vi "05TRM500_AnalyzeReceive_V2.vi"(5 "INC":dbl, 6 "Directory":path, 7 "MPH":dbl, 8 "error in (no error)":errorcluster, 10 "String":string, 11 "Enum":enum16{"Initialize", "Analyze"}(ring)) -> (0 "error out":errorcluster, 3 "Data":T1)   [LabVIEW 2020]
uses:
  <vilib>/regexp/Match Regular Expression.xnode
panel:
  out "File Ref":refnum<file>
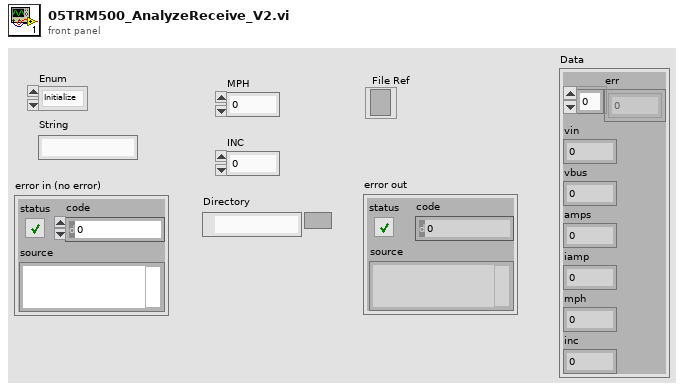
[diagram p1: front panel]
types:
  T1 = cluster{"err":i32[], "vin":i32, "vbus":i32, "amps":i32, "iamp":i32, "mph":i32, "inc":i32}
  T2 = enum16{"Initialize", "Next", "Send RSET", "Set MPH", "Set INC", "Part to 0"}
  T3 = enum16{"Initialize", "FootReceive", "FootDisplay"}
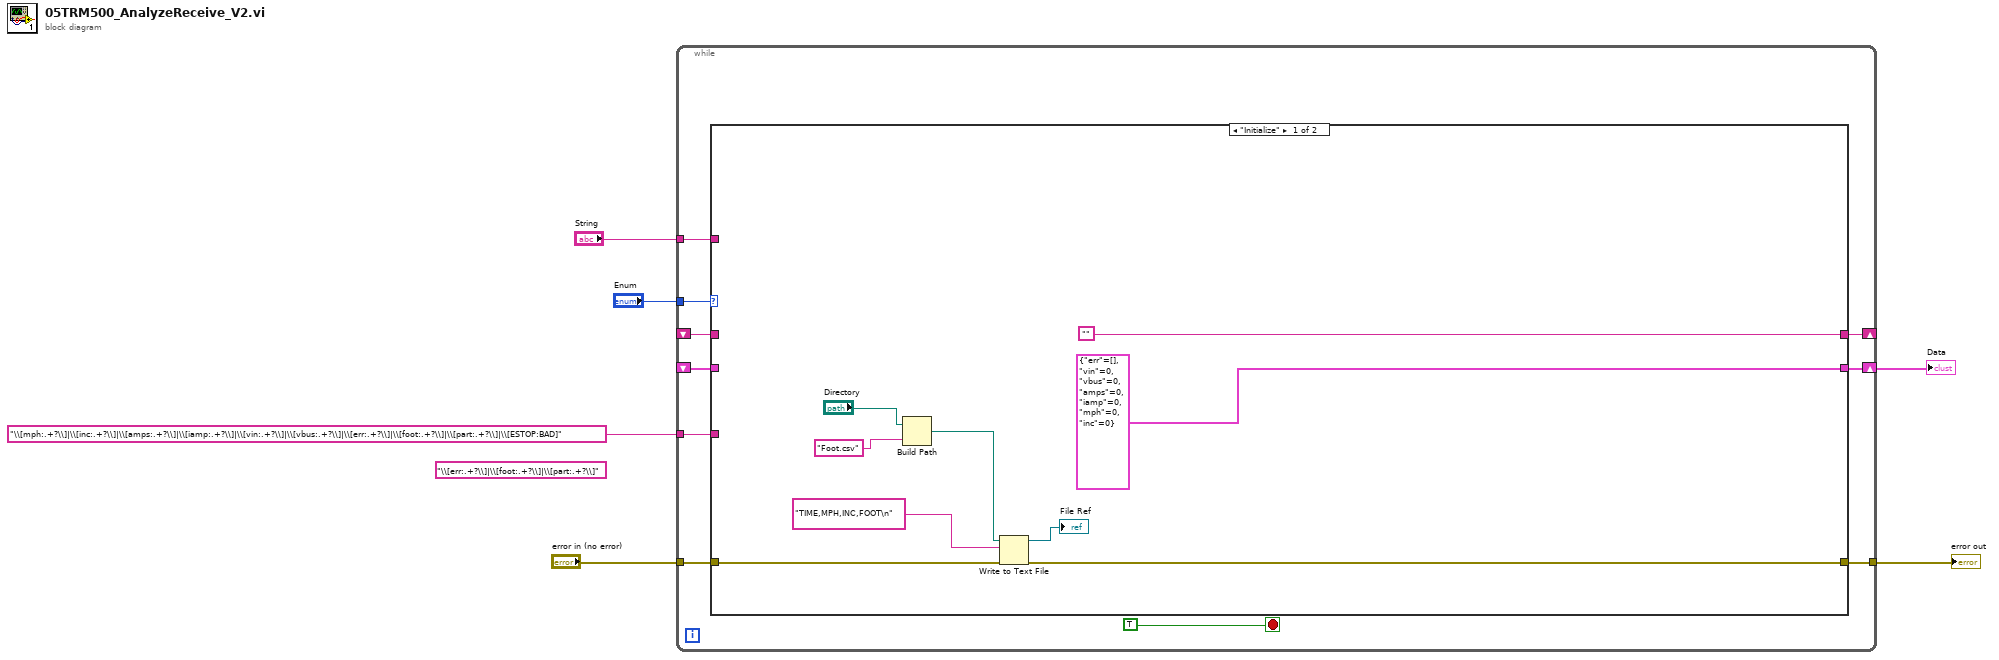
[diagram p0: block diagram]
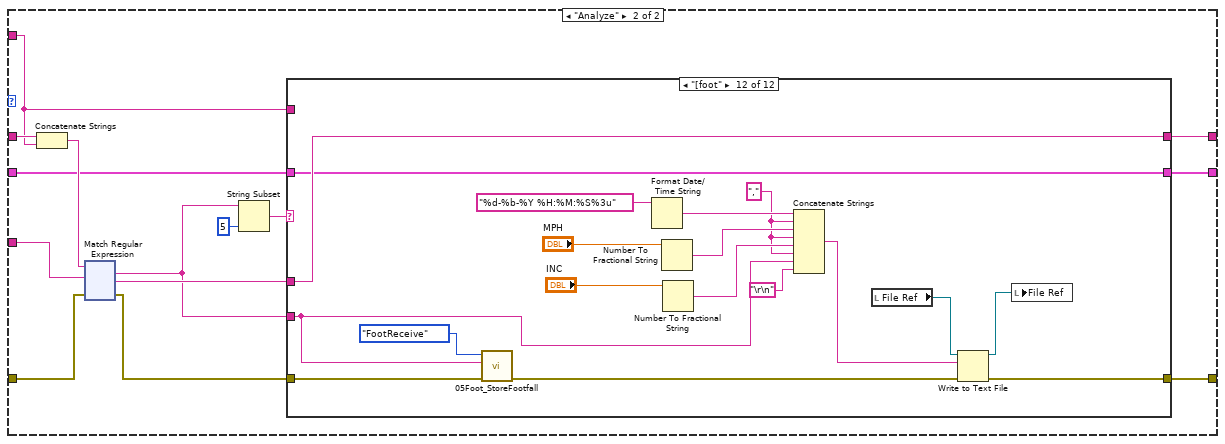
[diagram p2: hidden frame]
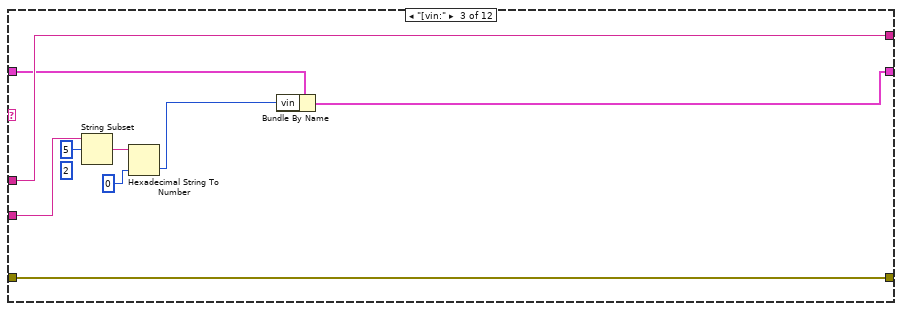
[diagram p5: hidden frame]
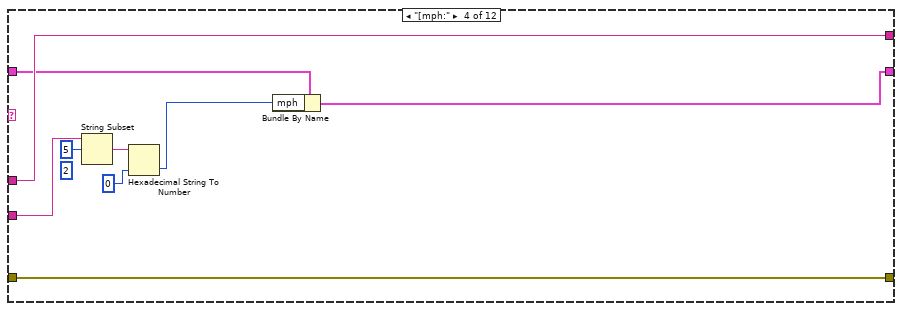
[diagram p6: hidden frame]
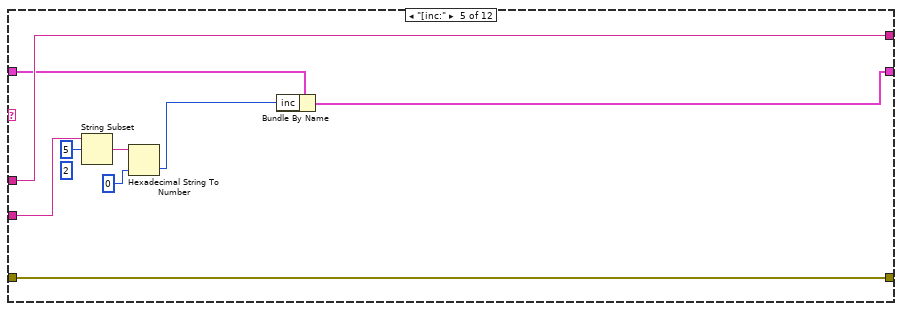
[diagram p7: hidden frame]
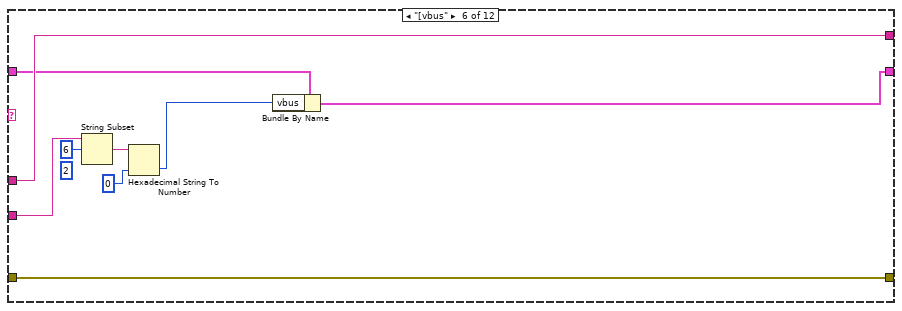
[diagram p8: hidden frame]
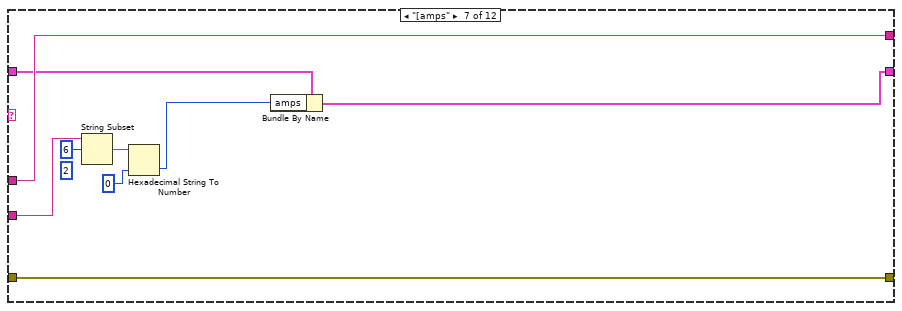
[diagram p9: hidden frame]
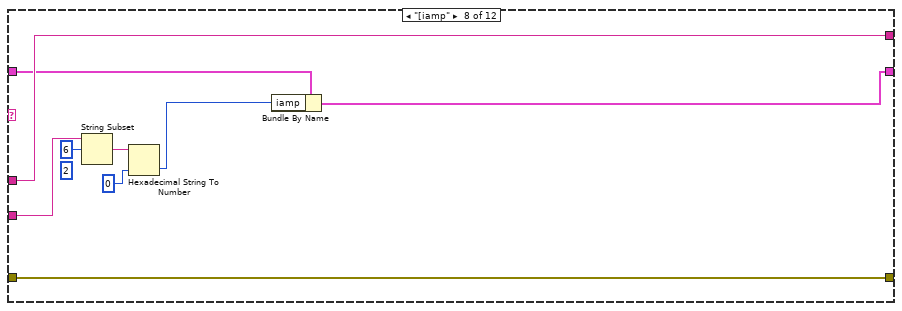
[diagram p10: hidden frame]
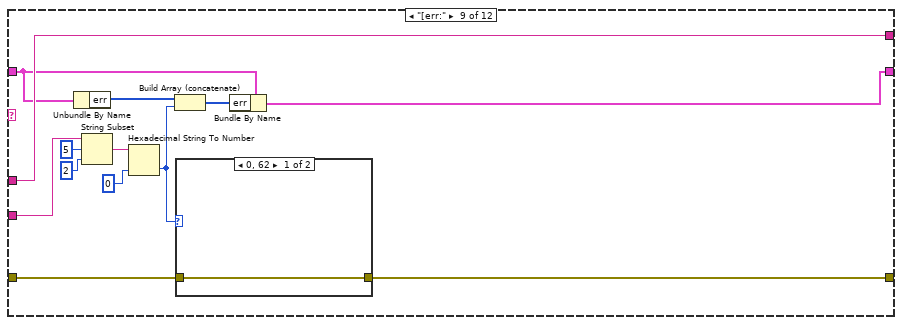
[diagram p11: hidden frame]
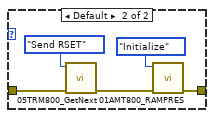
[diagram p12: hidden frame]
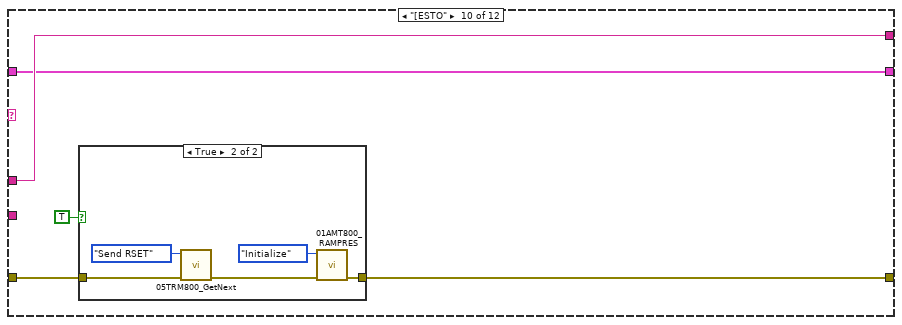
[diagram p13: hidden frame]
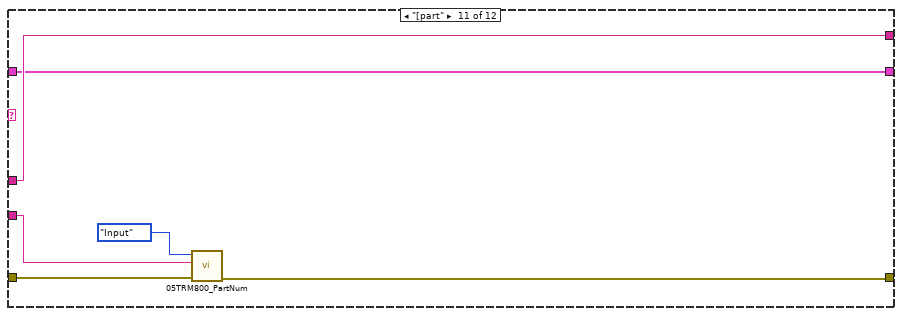
[diagram p15: hidden frame]
diagram:
  (unwired) "\\[err:.+?\\]|\\[foot:.+?\\]|\\[part:.+?\\]" ("regular expression")
  n1 = while {
    tunnel: "error in (no error)" -> [w13]
    tunnel: [w14] -> w5
    tunnel: "Enum" -> [w15]
    shift-right: [w12] -> _
    shift-left: _ -> [w11]
    tunnel: "String" -> [w10]
    tunnel: "\\[mph:.+?\\]|\\[inc:.+?\\]|\\[amps:.+?\\]|\\[iamp:.+?\\]|\\[vin:.+?\\]|\\[vbus:.+?\\]|\\[err:.+?\\]|\\[foot:.+?\\]|\\[part:.+?\\]|\\[ESTOP:BAD]" ("regular expression") -> [w9]
    shift-right: [w8] -> w1
    shift-left: _ -> [w7]
    stop <- TRUE stop-if-true
    n2 = case shown="\"Initialize\"" w15 {
      tunnel: [w20 w35] -> w14
      tunnel: w13 -> [w23 w32]
      tunnel: ["" w37] -> w12
      tunnel: w11 -> [_ w39]
      tunnel: w10 -> [_ w38]
      tunnel: w9 -> [_ w34]
      tunnel: [T1 {"err"=[], "vin"=0, "vbus"=0, "amps"=0, "iamp"=0, "mph"=0, "inc"=0} w26] -> w8
      tunnel: w7 -> [_ w27]
      frame "Initialize" {
        n3 = Build Path(base path="Directory", name or relative path="Foot.csv") -> (appended path=w17:path)
        n4 = Write to Text File(file (use dialog)=w17, text="TIME,MPH,INC,FOOT\n", error in=w23) -> (refnum out=→"File Ref":refnum<file>, error out=w20:errorcluster)  [unwired: 1 in, 1 out]
      }
      frame "Analyze" {
        n5 = Concatenate Strings(w39, w38) -> (w33:string)
        n6 = xnode "Match Regular Expression"("input string"=w33, "regular expression"=w34, "error in"=w32) -> ("whole match"=w28:string, "after match"=w36:string, "error out"=w31:errorcluster)  [unwired: 3 in, 2 out]
        n7 = String Subset(string=w28, length (rest)=5 ("length (rest)")) -> (substring=w30:string)  [unwired: 1 in]
        n8 = case shown="\"[foot\"" w30 {
          tunnel: w38 -> [w156 _ _ _ _ _ _ _ _ _ _ _]
          tunnel: [w156 w159 w168 w177 w186 w195 w204 w213 w226 w237 w249 w267] -> w37
          tunnel: w36 -> [_ w159 w168 w177 w186 w195 w204 w213 w226 w237 w249 w267]
          tunnel: [w155 w158 w160 w169 w178 w187 w196 w205 w216 w234 w247 w258] -> w35
          tunnel: w31 -> [w155 w158 w160 w169 w178 w187 w196 w205 w225 w236 w248 w266]
          tunnel: w28 -> [_ _ w164 w173 w182 w191 w200 w209 w221 _ w246 w257]
          tunnel: w27 -> [w154 w157 w163 w172 w181 w190 w199 w208 w218 w235 w244 w264]
          tunnel: [w154 w157 w162 w171 w180 w189 w198 w207 w217 w235 w244 w264] -> w26
          frame "" {
          }
          frame Default {
          }
          frame "[vin:" {
            (unwired) 2 ("length (rest)")
            n9 = String Subset(string=w164, offset (0)=5) -> (substring=w166:string)  [unwired: 1 in]
            n10 = Hexadecimal String To Number(string=w166, default (0uL)=0 ("default (0 U32)")) -> (number=w161:i32)  [unwired: 1 in, 1 out]
            n11 = Bundle By Name(cluster=w163, "vin"=w161) -> (w162:T1)
          }
          frame "[mph:" {
            (unwired) 2 ("length (rest)")
            n12 = String Subset(string=w173, offset (0)=5) -> (substring=w175:string)  [unwired: 1 in]
            n13 = Hexadecimal String To Number(string=w175, default (0uL)=0 ("default (0 U32)")) -> (number=w170:i32)  [unwired: 1 in, 1 out]
            n14 = Bundle By Name(cluster=w172, "mph"=w170) -> (w171:T1)
          }
          frame "[inc:" {
            (unwired) 2 ("length (rest)")
            n15 = String Subset(string=w182, offset (0)=5) -> (substring=w184:string)  [unwired: 1 in]
            n16 = Hexadecimal String To Number(string=w184, default (0uL)=0 ("default (0 U32)")) -> (number=w179:i32)  [unwired: 1 in, 1 out]
            n17 = Bundle By Name(cluster=w181, "inc"=w179) -> (w180:T1)
          }
          frame "[vbus" {
            (unwired) 2 ("length (rest)")
            n18 = String Subset(string=w191, offset (0)=6) -> (substring=w193:string)  [unwired: 1 in]
            n19 = Hexadecimal String To Number(string=w193, default (0uL)=0 ("default (0 U32)")) -> (number=w188:i32)  [unwired: 1 in, 1 out]
            n20 = Bundle By Name(cluster=w190, "vbus"=w188) -> (w189:T1)
          }
          frame "[amps" {
            (unwired) 2 ("length (rest)")
            n21 = String Subset(string=w200, offset (0)=6) -> (substring=w202:string)  [unwired: 1 in]
            n22 = Hexadecimal String To Number(string=w202, default (0uL)=0 ("default (0 U32)")) -> (number=w197:i32)  [unwired: 1 in, 1 out]
            n23 = Bundle By Name(cluster=w199, "amps"=w197) -> (w198:T1)
          }
          frame "[iamp" {
            (unwired) 2 ("length (rest)")
            n24 = String Subset(string=w209, offset (0)=6) -> (substring=w211:string)  [unwired: 1 in]
            n25 = Hexadecimal String To Number(string=w211, default (0uL)=0 ("default (0 U32)")) -> (number=w206:i32)  [unwired: 1 in, 1 out]
            n26 = Bundle By Name(cluster=w208, "iamp"=w206) -> (w207:T1)
          }
          frame "[err:" {
            n27 = Unbundle By Name(w218) -> ("err"=w220:i32[])
            n28 = String Subset(string=w221, offset (0)=5, length (rest)=2 ("length (rest)")) -> (substring=w222:string)
            n29 = Hexadecimal String To Number(string=w222, default (0uL)=0 ("default (0 U32)")) -> (number=w214:i32)  [unwired: 1 in, 1 out]
            n30 = Build Array (concatenate)(w220, w214) -> (w219:i32[])
            n31 = case shown="0, 62" w214 {
              tunnel: w225 -> [w227 w232]
              tunnel: [w227 w229] -> w216
              frame 0, 62 {
              }
              frame Default {
                n32 = call "05TRM800_GetNext.vi"("error in (no error)"=w232, "Enum"=T2."Send RSET") -> ("error out"=w230:errorcluster)  [unwired: 8 in, 1 out]
                n33 = call "01AMT800_RAMPRES.vi"("error in (no error)"=w230, "Enum"=enum16{"Initialize", "Set"}."Initialize") -> ("error out"=w229:errorcluster)  [unwired: 7 in, 2 out]
              }
            }
            n34 = Bundle By Name(cluster=w218, "err"=w219) -> (w217:T1)
          }
          frame "[ESTO" {
            n35 = case shown="True" TRUE {
              tunnel: w236 -> [w238 w243]
              tunnel: [w238 w239] -> w234
              frame False {
              }
              frame True {
                n36 = call "05TRM800_GetNext.vi"("error in (no error)"=w243, "Enum"=T2."Send RSET") -> ("error out"=w240:errorcluster)  [unwired: 8 in, 1 out]
                n37 = call "01AMT800_RAMPRES.vi"("error in (no error)"=w240, "Enum"=enum16{"Initialize", "Set"}."Initialize") -> ("error out"=w239:errorcluster)  [unwired: 7 in, 2 out]
              }
            }
          }
          frame "[part" {
            n38 = call "05TRM800_PartNum.vi"("error in (no error)"=w248, "Input"=w246, "Enum"=enum16{"Initialize", "Get", "Input"}."Input") -> ("error out"=w247:errorcluster)  [unwired: 7 in, 1 out]
          }
          frame "[foot" {
            w255 = ","
            n39 = call "05Foot_StoreFootfall.vi"("error in (no error)"=w266, "FootIn"=w257, "Enum"=T3."FootReceive") -> ("error out"=w259:errorcluster)  [unwired: 7 in, 1 out]
            n40 = Format Date/Time String(time format string (%c)="%d-%b-%Y %H:%M:%S%3u") -> (date/time string=w262:string)  [unwired: 2 in]
            n41 = Number To Fractional String(number="MPH") -> (F-format string=w261:string)  [unwired: 3 in]
            n42 = Number To Fractional String(number="INC") -> (F-format string=w260:string)  [unwired: 3 in]
            n43 = Concatenate Strings(w262, w255, w261, w255, w260, w255, w257, "\r\n") -> (w256:string)
            n44 = local read "File Ref"() -> (w253:refnum<file>)
            n45 = Write to Text File(file (use dialog)=w253, text=w256, error in=w259) -> (refnum out=w252:refnum<file>, error out=w258:errorcluster)  [unwired: 1 in, 1 out]
            n46 = local write "File Ref"(w252) -> ()
          }
        }
      }
    }
  }
  "error out" <- w5
  "Data" <- w1
